vi "runFirstState.vi"(6 "Fault?":bool, 7 "Ready":bool, 8 "error in (no error)":errorcluster, 9 "Actuators in":T1, 10 "State in":T2, 11 "RunType in":refnum<class "RunType.lvclass">) -> (0 "error out":errorcluster, 1 "Actuators out":T1, 2 "State out":T2, 3 "RunType out":refnum<class "RunType.lvclass">)   [LabVIEW 2017, in "ControlLibrary.lvlib" / "RunType.lvclass"]
uses:
  RunType.lvclass
  TypeDef_ControlState.ctl
  TypeDef_DigitalOuts.ctl
  TypeDef_RunParameters.ctl
  RunType.lvclass/RunType.ctl
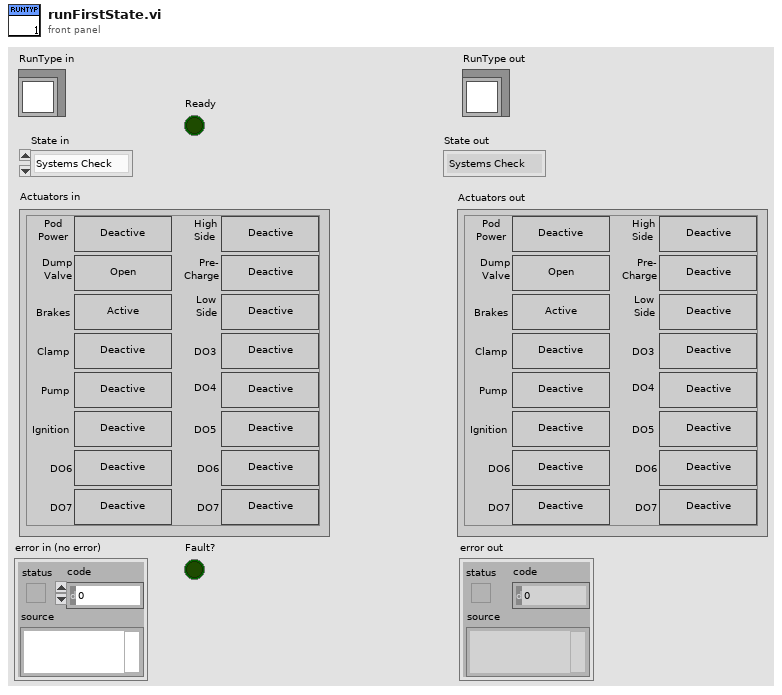
[diagram p1: front panel]
types:
  T1 = typedef "TypeDef_DigitalOuts.ctl" = cluster{"Pod Power":bool, "Dump Valve":bool, "Brakes":bool, "Clamp":bool, "Pump":bool, "Ignition":bool, "DO6":bool, "DO7":bool, "HighSide":bool, "Precharge":bool, "LowSide":bool, "DO3":bool, "DO4":bool, "DO5":bool, "DO62":bool, "DO72":bool}
  T2 = typedef "TypeDef_ControlState.ctl" = enum16{"Systems Check", "Idle", "Ready", "Pushing", "Coast", "Braking", "Fault", "Shutdown", "Service", "Precharge", "Blank"}
  T3 = typedef "TypeDef_RunParameters.ctl" = cluster{"Distance Threshold (ft)":dbl, "Time Threshold (s)":dbl, "Target (I16)":i16}
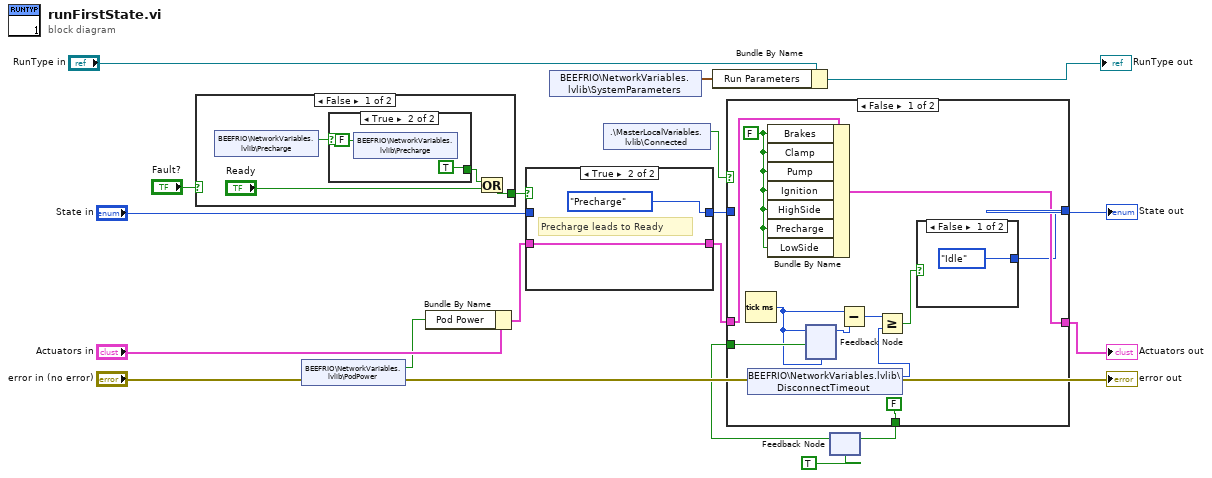
[diagram p0: block diagram]
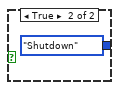
[diagram p2: hidden frame]
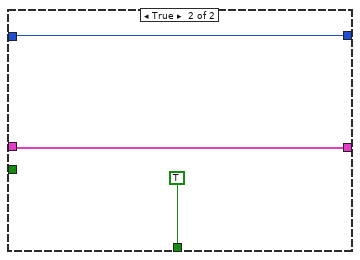
[diagram p3: hidden frame]
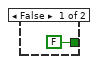
[diagram p5: hidden frame]
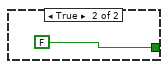
[diagram p6: hidden frame]
diagram:
  n1 = case shown="False" "Fault?" {
    tunnel: [w22 FALSE ("Ready")] -> w8
    frame False {
      n2 = shared-variable "BEEFRIO\\NetworkVariables.lvlib\\Precharge"() -> (w23:bool)  [unwired: 1 in, 1 out]
      n3 = case shown="True" w23 {
        tunnel: [FALSE TRUE] -> w20
        frame False {
        }
        frame True {
          n4 = shared-variable "BEEFRIO\\NetworkVariables.lvlib\\Precharge"(FALSE ("Precharge")) -> ()  [unwired: 1 in, 1 out]
        }
      }
      n5 = Or(x=w20, y="Ready") -> (x .or. y?=w22:bool)
    }
    frame True {
    }
  }
  n6 = shared-variable "BEEFRIO\\NetworkVariables.lvlib\\PodPower"(error in="error in (no error)") -> (w10:bool, error out=→"error out":errorcluster)
  n7 = Bundle By Name(cluster="Actuators in", "Pod Power"=w10) -> (w7:T1)
  n8 = case shown="True" w8 {
    tunnel: [w29 TypeDef_ControlState."Precharge" ("State in")] -> w5
    tunnel: "State in" -> [w29 _]
    tunnel: w7 -> [w28 w30]
    tunnel: [w28 w30] -> w4
    frame False {
    }
    frame True {
      # "Precharge leads to Ready"
    }
  }
  n9 = shared-variable "BEEFRIO\\NetworkVariables.lvlib\\SystemParameters"() -> (w11:T3)  [unwired: 1 in, 1 out]
  n10 = shared-variable ".\\MasterLocalVariables.lvlib\\Connected"() -> (w6:bool)  [unwired: 1 in, 1 out]
  n11 = Bundle By Name(cluster="RunType in", "Run Parameters"=w11) -> (→"RunType out":refnum<class "RunType.lvclass">)
  n12 = feedback #1(TRUE) -> (w3:bool)
  n13 = case shown="False" w6 {
    tunnel: [w39 w47] -> w15
    tunnel: w5 -> [_ w47]
    tunnel: [w41 w46] -> w12
    tunnel: w4 -> [w42 w46]
    tunnel: w3 -> [w38 _]
    tunnel: [FALSE TRUE] -> w1
    frame False {
      w40 = FALSE ("Brakes")
      n14 = Tick Count (ms)() -> (millisecond timer value=w35:u32)
      n15 = shared-variable "BEEFRIO\\NetworkVariables.lvlib\\DisconnectTimeout"() -> (w32:u32)  [unwired: 1 in, 1 out]
      n16 = Bundle By Name(cluster=w42, "Brakes"=w40, "Clamp"=w40, "Pump"=w40, "Ignition"=w40, "HighSide"=w40, "Precharge"=w40, "LowSide"=w40) -> (w41:T1)
      n17 = feedback-in #2(w35, w38) -> ()
      n18 = feedback #2(w35) -> (w36:u32)
      n19 = Subtract(x=w35, y=w36) -> (x-y=w34:u32)
      n20 = Greater Or Equal?(x=w34, y=w32) -> (x >= y?=w33:bool)
      n21 = case shown="False" w33 {
        tunnel: [TypeDef_ControlState."Idle" ("State in") TypeDef_ControlState."Shutdown" ("State in")] -> w39
        frame False {
        }
        frame True {
        }
      }
    }
    frame True {
    }
  }
  "State out" <- w15
  "Actuators out" <- w12
  n22 = feedback-in #1(w1) -> ()
